vi "Atividade 2.vi"() -> ()   [LabVIEW 2015]
panel:
  in  "d":bool
  in  "c":bool
  in  "e":bool
  in  "g":bool
  in  "b":bool
  in  "f":bool
  in  "a":bool
  out "c":bool
  out "d":bool
  out "e":bool
  out "b":bool
  out "g":bool
  out "f":bool
  out "a":bool
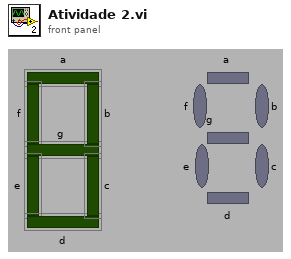
[diagram p1: front panel]
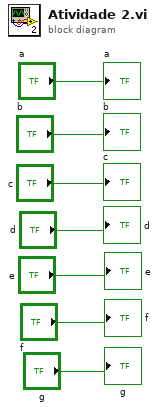
[diagram p0: block diagram]
diagram:
  "a" <- "a"
  "f" <- "f"
  "g" <- "g"
  "b" <- "b"
  "e" <- "e"
  "d" <- "d"
  "c" <- "c"
